vi "POBOTS_RobotDriveArcadeDrive_Standard(NoSaturation).vi"(6 "Mult":dbl, 7 "Positive":bool, 8 "error in (no error)":errorcluster, 9 "Y axis value":dbl, 10 "X axis value":dbl, 11 "RobotDriveDevRef":T1={"DevStatus"={"status"=FALSE, "code"=0, "source"=""}, "Motors[]"=[], "Square Inputs"=FALSE, "Max Output"=1.0, "Isochronous"=FALSE}) -> (0 "error out":errorcluster, 2 "Motor Values":dbl[](array[numeric]), 3 "RobotDriveDevRef":T1={"DevStatus"={"status"=FALSE, "code"=0, "source"=""}, "Motors[]"=[], "Square Inputs"=FALSE, "Max Output"=1.0, "Isochronous"=FALSE})   [LabVIEW 2013]
doc: "Uses a standard algorithm to configure the motors for arcade driving. This algorithm does not saturate over half of the range.\n\nThis software is licensed. Open the labview\\readme\\WPI Robotics Library Open Source License.txt file for more information."
uses:
  <vilib>/Rock Robotics/WPI/RobotDrive/WPI_RobotDriveDevRef.ctl
  <vilib>/Rock Robotics/WPI/MotorControl/WPI_MotorControlDeviceRef.ctl
  <vilib>/Rock Robotics/SystemInterfaces/Typedef/FPGA_TypedefDigitalModule.ctl
  <vilib>/Rock Robotics/SystemInterfaces/DIO/FPGA_DIOPWMChannel.ctl
  <vilib>/Rock Robotics/WPI/PWM/WPI_PWMDeadband.ctl
  <vilib>/Rock Robotics/WPI/CAN/Jaguar/SubVIs/WPI_CANJaguar_ControlMode.ctl
  <vilib>/Rock Robotics/WPI/PWM/WPI_PWMTransform_ConPane.ctl
  <vilib>/Rock Robotics/SystemInterfaces/NetworkCommunication/NetComm_UsageReport_ResourceType.ctl
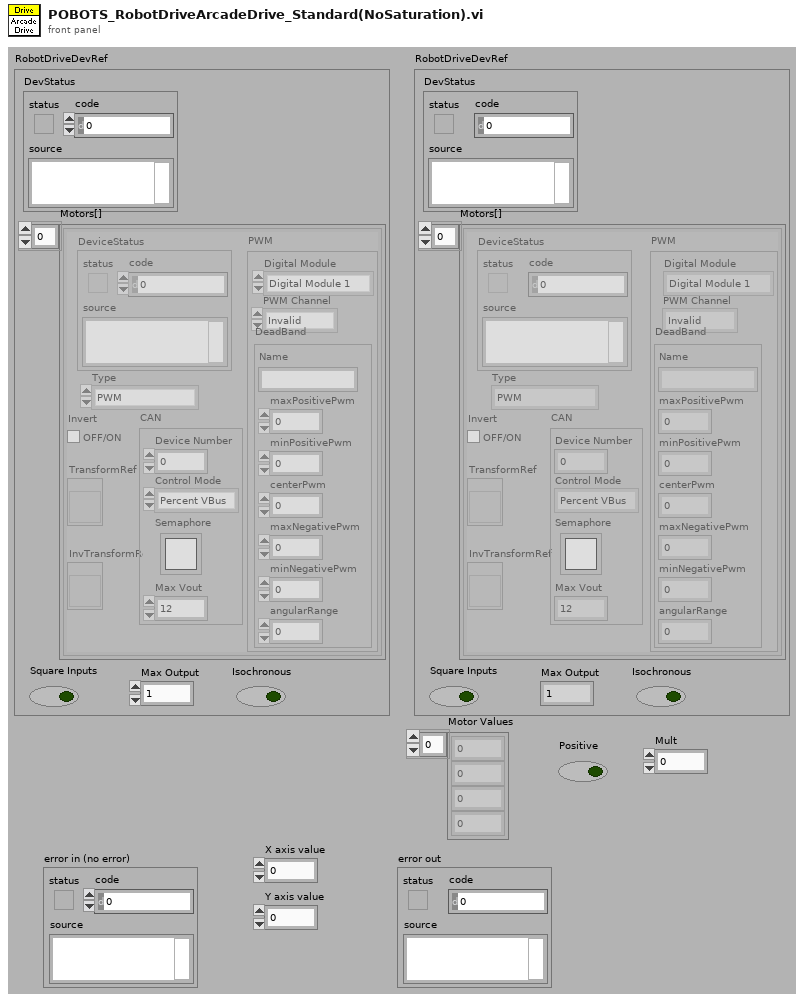
[diagram p1: front panel]
types:
  T1 = typedef "WPI_RobotDriveDevRef.ctl" = cluster{"DevStatus":errorcluster, "Motors[]":T2[], "Square Inputs":bool, "Max Output":dbl, "Isochronous":bool}
  T2 = typedef "WPI_MotorControlDeviceRef.ctl" = cluster{"DeviceStatus":errorcluster, "Type":enum16{"PWM", "CAN"}, "PWM":cluster{"Digital Module":T3, "PWM Channel":T4, "DeadBand":T5}, "CAN":cluster{"Device Number":u8, "Control Mode":T6, "Semaphore":T7, "Max Vout":dbl}, "Invert":bool, "TransformRef":T8, "InvTransformRef":T8}
  T3 = typedef "FPGA_TypedefDigitalModule.ctl" = enum16{"Digital Module 1", "Digital Module 2"}
  T4 = typedef "FPGA_DIOPWMChannel.ctl" = enum8{"PWM 1", "PWM 2", "PWM 3", "PWM 4", "PWM 5", "PWM 6", "PWM 7", "PWM 8", "PWM 9", "PWM 10", "Invalid"}
  T5 = typedef "WPI_PWMDeadband.ctl" = cluster{"Name":string, "maxPositivePwm":i32, "minPositivePwm":i32, "centerPwm":i32, "maxNegativePwm":i32, "minNegativePwm":i32, "angularRange":u16}
  T6 = typedef "WPI_CANJaguar_ControlMode.ctl" = enum8{"Percent VBus", "Current", "Speed", "Position", "Voltage"}
  T7 = typedef "Semaphore RefNum" = refnum<k1>
  T8 = typedef "WPI_PWMTransform_ConPane.ctl" = refnum<vi>
  T9 = typedef "NetComm_UsageReport_ResourceType.ctl" = enum8{"Controller", "Module", "Language", "CANPlugin", "Accelerometer", "ADXL345", "AnalogChannel", "AnalogTrigger", "AnalogTriggerOutput", "CANJaguar", "Compressor", "Counter", "Dashboard", "DigitalInput", "DigitalOutput", "DriverStationCIO", "DriverStationEIO", "DriverStationLCD", "Encoder", "GearTooth", "Gyro", "I2C", "Framework", "Jaguar", "Joystick", "Kinect", "KinectStick", "PIDController", "Preferences", "PWM", "Relay", "RobotDrive", "SerialPort", "Servo", "Solenoid", "SPI", "Task", "Ultrasonic", "Victor", "Button", "Command", "AxisCamera", "PCVideoServer", "SmartDashboard", "Talon", "HiTechnicColorSensor", "HiTechnicAccel", "HiTechnicCompass", "SRF08"}
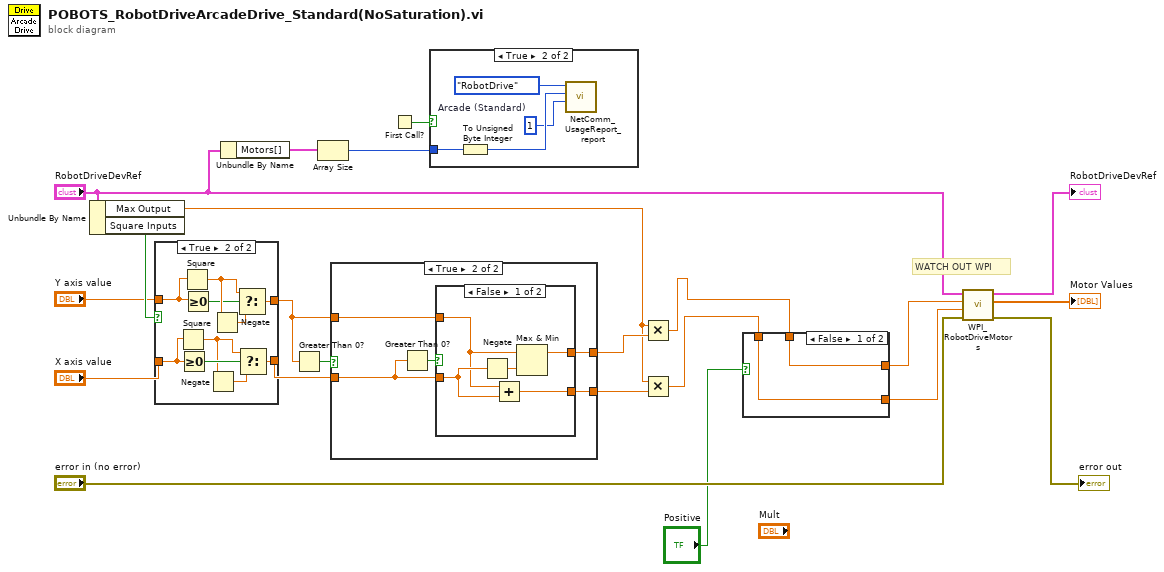
[diagram p0: block diagram]
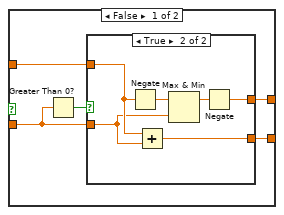
[diagram p4: hidden frame]
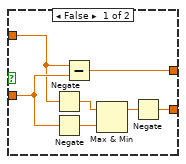
[diagram p5: hidden frame]
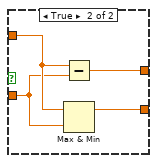
[diagram p6: hidden frame]
diagram:
  # "WATCH OUT WPI"
  n1 = Unbundle By Name("RobotDriveDevRef") -> ("Max Output"=w13:dbl, "Square Inputs"=w21:bool)
  n2 = case shown="True" w21 {
    tunnel: [w23 w34] -> w18
    tunnel: [w24 w33] -> w19
    tunnel: "X axis value" -> [w23 w32]
    tunnel: "Y axis value" -> [w24 w31]
    frame False {
    }
    frame True {
      n3 = Square(x=w32) -> (x^2=w29:dbl)
      n4 = Greater Or Equal To 0?(x=w32) -> (x >= 0?=w30:bool)
      n5 = Square(x=w31) -> (x^2=w26:dbl)
      n6 = Greater Or Equal To 0?(x=w31) -> (x >= 0?=w25:bool)
      n7 = Negate(x=w29) -> (-x=w28:dbl)
      n8 = Negate(x=w26) -> (-x=w27:dbl)
      n9 = Select(t=w26, s=w25, f=w27) -> (s? t:f=w33:dbl)
      n10 = Select(t=w29, s=w30, f=w28) -> (s? t:f=w34:dbl)
    }
  }
  n11 = Unbundle By Name("RobotDriveDevRef") -> ("Motors[]"=w8:T2[])
  n12 = Greater Than 0?(x=w19) -> (x > 0?=w20:bool)
  n13 = Array Size(array=w8) -> (size(s)=w7:i32)
  n14 = case shown="True" w20 {
    tunnel: w18 -> [w38 w56]
    tunnel: w19 -> [w37 w55]
    tunnel: [w36 w54] -> w17
    tunnel: [w35 w53] -> w14
    frame False {
      n15 = Greater Than 0?(x=w38) -> (x > 0?=w39:bool)
      n16 = case shown="True" w39 {
        tunnel: w38 -> [w46 w48]
        tunnel: w37 -> [w44 w49]
        tunnel: [w40 w50] -> w36
        tunnel: [w41 w47] -> w35
        frame False {
          n17 = Negate(x=w44) -> (-x=w45:dbl)
          n18 = Negate(x=w46) -> (-x=w43:dbl)
          n19 = Subtract(x=w44, y=w46) -> (x-y=w40:dbl)
          n20 = Max & Min(x=w45, y=w43) -> (max(x,y)=w42:dbl)  [unwired: 1 out]
          n21 = Negate(x=w42) -> (-x=w41:dbl)
        }
        frame True {
          n22 = Negate(x=w49) -> (-x=w52:dbl)
          n23 = Add(x=w49, y=w48) -> (x+y=w47:dbl)
          n24 = Max & Min(x=w52, y=w48) -> (max(x,y)=w51:dbl)  [unwired: 1 out]
          n25 = Negate(x=w51) -> (-x=w50:dbl)
        }
      }
    }
    frame True {
      n26 = Greater Than 0?(x=w56) -> (x > 0?=w57:bool)
      n27 = case shown="False" w57 {
        tunnel: w56 -> [w62 w64]
        tunnel: w55 -> [w59 w65]
        tunnel: [w60 w63] -> w54
        tunnel: [w58 w66] -> w53
        frame False {
          n28 = Negate(x=w62) -> (-x=w61:dbl)
          n29 = Add(x=w59, y=w62) -> (x+y=w58:dbl)
          n30 = Max & Min(x=w59, y=w61) -> (max(x,y)=w60:dbl)  [unwired: 1 out]
        }
        frame True {
          n31 = Subtract(x=w65, y=w64) -> (x-y=w63:dbl)
          n32 = Max & Min(x=w65, y=w64) -> (max(x,y)=w66:dbl)  [unwired: 1 out]
        }
      }
    }
  }
  n33 = First Call?() -> (First Call?: T/F=w10:bool)
  n34 = case shown="True" w10 {
    tunnel: w7 -> [_ w69]
    frame False {
    }
    frame True {
      w67 = u8 1  # Arcade (Standard)
      n35 = To Unsigned Byte Integer(number=w69) -> (unsigned 8bit integer=w68:u8)
      n36 = call <vilib>:"NetComm_UsageReport_report.vi"("Context"=w67, "Instance Number"=w68, "Resource Type"=NetComm_UsageReport_ResourceType."RobotDrive") -> ()  [unwired: 9 in]
    }
  }
  n37 = Multiply(x=w13, y=w17) -> (x*y=w3:dbl)
  n38 = Multiply(x=w13, y=w14) -> (x*y=w1:dbl)
  n39 = case shown="False" "Positive" {
    tunnel: [w71 w74] -> w4
    tunnel: w3 -> [w71 w74]
    tunnel: [w72 w73] -> w2
    tunnel: w1 -> [w72 w73]
    frame False {
    }
    frame True {
    }
  }
  n40 = call <vilib>:"WPI_RobotDriveMotors.vi"("error in (no error)"="error in (no error)", "RightSpeed"=w2, "LeftSpeed"=w4, "RobotDriveDevRef"="RobotDriveDevRef") -> ("error out"=→"error out":errorcluster, "Motor Values"=→"Motor Values":dbl[], "RobotDriveDevRef"=→"RobotDriveDevRef":T1)  [unwired: 5 out]
